vi "add_rate.vi"(1 "Rate array in":dbl[](array[numeric]), 2 "Polarization array":dbl[](array[numeric]), 3 "Eventnum array":i64[](array[numeric]), 4 "Array position":i32) -> (0 "Rate array out":dbl[](array[numeric]))   [LabVIEW 2015]
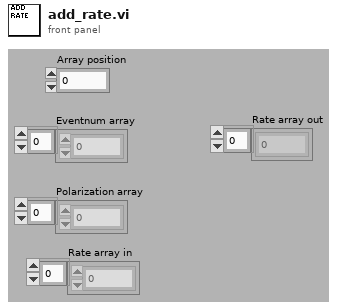
[diagram p1: front panel]
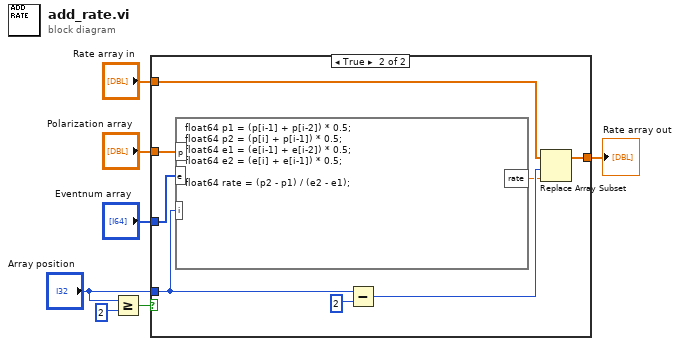
[diagram p0: block diagram]
diagram:
  n1 = Greater Or Equal?(x="Array position", y=2) -> (x >= y?=w7:bool)
  n2 = case shown="True" w7 {
    tunnel: "Rate array in" -> [w8 w15]
    tunnel: [w8 w14] -> w2
    tunnel: "Array position" -> [_ w16]
    tunnel: "Polarization array" -> [_ w13]
    tunnel: "Eventnum array" -> [_ w12]
    frame False {
    }
    frame True {
      n3 = formula code="float64 p1 = (p[i-1] + p[i-2]) * 0.5;\nfloat64 p2 = (p[i] + p[i-1]) * 0.5;\nfloat64 e1 = (e[i-1] + e[i-2]) * 0.5;\nfloat64 e2 = (e[i] + e[i-1]) * 0.5;\n\nfloat64 rate = (p2 - p1) / (e2 - e1);"("p"=w13, "e"=w12, "i"=w16) -> ("rate"=w9:dbl)
      n4 = Subtract(x=w16, y=2) -> (x-y=w11:i32)
      n5 = Replace Array Subset(array=w15, new element=w9, index=w11) -> (w14:dbl[])
    }
  }
  "Rate array out" <- w2
